vi "Read System Name.vi"(8 "error in":errorcluster, 11 "cRIO in":refnum<class "cRIO.lvclass">) -> (0 "error out":errorcluster, 2 "system name":string, 3 "cRIO out":refnum<class "cRIO.lvclass">)   [LabVIEW 2015, in "cRIO.lvclass"]
uses:
  cRIO.lvclass
  cRIO.lvclass/cRIO.ctl
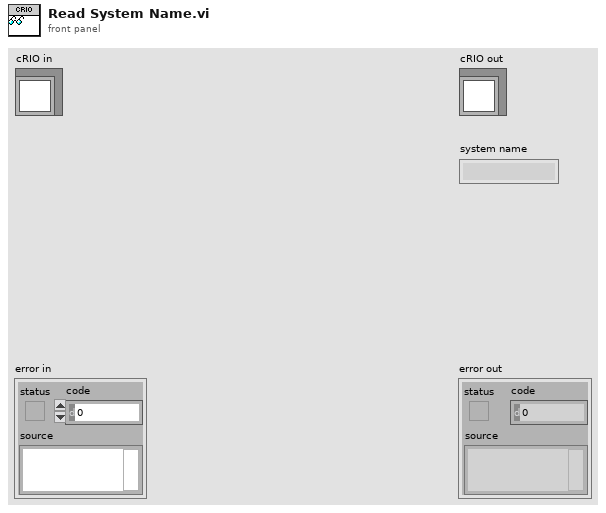
[diagram p1: front panel]
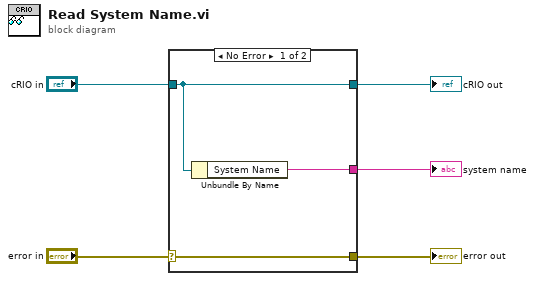
[diagram p0: block diagram]
diagram:
  n1 = case shown="No Error" "error in" {
    selector: "error in" -> [w8 w9]
    tunnel: [w8 w9] -> w4
    tunnel: [w7 w10] -> w2
    tunnel: "cRIO in" -> [w7 w10]
    tunnel: [w6 _] -> w1
    frame No Error {
      n2 = Unbundle By Name(w7) -> ("System Name"=w6:string)
    }
    frame Error {
    }
  }
  "error out" <- w4
  "cRIO out" <- w2
  "system name" <- w1
